vi "Finalize Spawn.vi"(7 "Actor in":refnum<data-value>, 8 "Error in":errorcluster, 10 "Attributes":refnum<data-value>) -> (0 "Error out":errorcluster, 5 "Actor out":refnum<data-value>)   [LabVIEW 2020, in "jettl.lvlib"]
uses:
  jettl.lvlib
  Msg/Msg.lvclass
  Actor/Actor.lvclass
  Msg Input/Msg Input.lvclass
  Msg Output/Msg Output.lvclass
  Msg Set.ctl
  Refs/Refs.lvclass
  Actor.ctl
  Unified Actor.ctl
  Unified Actor Relation.ctl
  Teller.ctl
  Msg.ctl
  Msgs.ctl
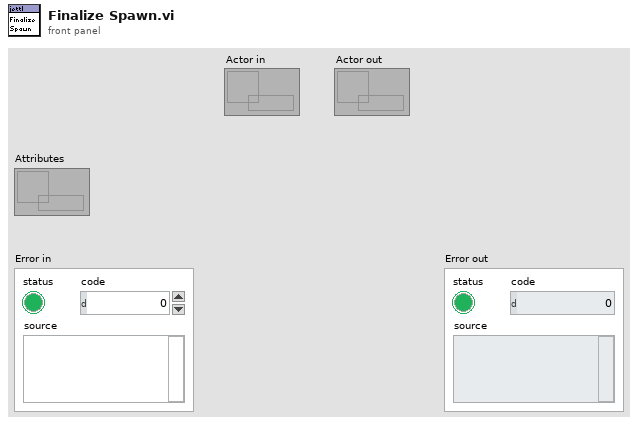
[diagram p1: front panel]
types:
  T1 = typedef "jettl.lvlib/Actor.ctl" = cluster{"Msgs":T2, "Leaf":bool, "Index":i32, "Actor":refnum<class "Actor.lvclass">, "Refs":refnum<class "Refs.lvclass">}
  T2 = typedef "jettl.lvlib/Msgs.ctl" = cluster{"Inbound":T3, "Outbound":T3, "Implemented":T3, "Tell Init":T3, "Tell Init Self":T3, "Tell Init Parent":T3, "Tell Init Child":T3, "Tell Forward":T3, "Tell Forward Self":T3, "Tell Forward Parent":T3, "Tell Forward Child":T3}
  T3 = typedef "jettl.lvlib/Msg Set.ctl" = set{refnum<class "Msg.lvclass">}
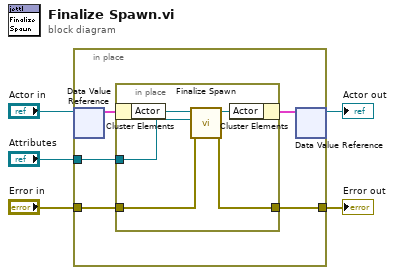
[diagram p0: block diagram]
diagram:
  n1 = in-place {
    in-place-border: "Attributes" -> [w8]
    in-place-border: "Error in" -> [w7]
    in-place-border: [w6] -> w1
    n2 = in-place-dvr #1("Actor in") -> (w10:T1)  [unwired: 1 out]
    n3 = in-place {
      in-place-border: w8 -> [w13]
      in-place-border: w7 -> [w12]
      in-place-border: [w11] -> w6
      n4 = in-place-cluster #2(w10) -> ("Actor"=w15:refnum<class "Actor.lvclass">)
      n5 = call-dynamic "Finalize Spawn.vi"("Error in"=w12, "Attributes"=w13, "Actor in"=w15) -> ("Error out"=w11:errorcluster, "Actor out"=w14:refnum<class "Actor.lvclass">)  [unwired: 7 in]
      n6 = in-place-cluster #2("Actor"=w14) -> (w9:T1)
    }
    n7 = in-place-dvr #1(w9) -> (→"Actor out":refnum<data-value>)  [unwired: 1 out]
  }
  "Error out" <- w1
